vi "Zservo.vi"() -> ()   [LabVIEW 2014]
uses:
  <vilib>/Instr/_visa.llb/VISA Configure Serial Port (Instr).vi
panel:
  in  "position":u8(slide) scale=0.0..254.0
  in  "stop":bool
  # "Pololu Maestro 6"
  # "SSC Servo \nControl Example"
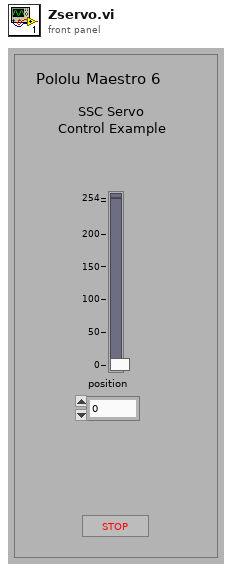
[diagram p1: front panel]
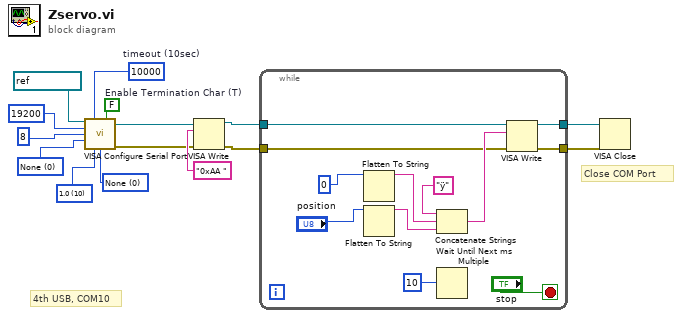
[diagram p0: block diagram]
diagram:
  w5 = u16 0 items=["None"=0, "XON/XOFF"=1, "RTS/CTS"=2, "DTR/DSR"=4] ("flow control")
  w6 = u16 10 items=["1.0"=10, "1.5"=15, "2.0"=20] ("stop bits")
  w7 = u16 0 items=["None", "Odd", "Even", "Mark", "Space"] ("parity")
  w11 = FALSE  # Enable Termination Char (T)
  w12 = u32 10000  # timeout (10sec)
  # "4th USB, COM10"
  # "Close COM Port"
  n1 = call-poly "VISA Configure Serial Port"("VISA resource name"=refnum<visa-resource-name> "COM10", "timeout (10sec)"=w12, "Enable Termination\nChar (T)"=w11, "baud rate (9600)"=u32 19200 ("baud rate"), "data bits (8)"=u16 8 ("data bits"), "parity (0:none)"=w7, "stop bits (10: 1 bit)"=w6, "flow control (0:none)"=w5) -> ("VISA resource name out"=w3:refnum<visa-resource-name>, "error out"=w4:errorcluster)  [unwired: 1 in, 5 out]
  n2 = VISA Write(VISA resource name=w3, write buffer="0xAA ", error in (no error)=w4) -> (VISA resource name out=w14:refnum<visa-resource-name>, error out=w13:errorcluster)  [unwired: 1 out]
  n3 = while {
    tunnel: w14 -> [w23]
    tunnel: w13 -> [w22]
    tunnel: [w18] -> w2
    tunnel: [w17] -> w1
    stop <- "stop" stop-if-true
    n4 = Flatten To String(anything=u16 0 ("data bits")) -> (data string=w26:string)  [unwired: 1 in, 4 out]
    n5 = Flatten To String(anything="position") -> (data string=w25:string)  [unwired: 1 in, 4 out]
    n6 = Concatenate Strings("ÿ", w26, w25) -> (w24:string)
    n7 = Wait Until Next ms Multiple(millisecond multiple=10) -> ()  [unwired: 1 out]
    n8 = VISA Write(VISA resource name=w23, write buffer=w24, error in (no error)=w22) -> (VISA resource name out=w18:refnum<visa-resource-name>, error out=w17:errorcluster)  [unwired: 1 out]
  }
  n9 = VISA Close(VISA resource name=w2, error in (no error)=w1) -> ()  [unwired: 1 out]
